vi "AudioStreamer.Initialize.vi"(1 "visible":bool) -> (0 "success":bool)   [LabVIEW 2020]
uses:
  <vilib>/Utility/sysdir.llb/System Directory Type.ctl
  <vilib>/Utility/config.llb/Read Key (I32).vi
  <vilib>/Utility/config.llb/NI_LVConfig.lvlib
panel:
  out "error out":errorcluster
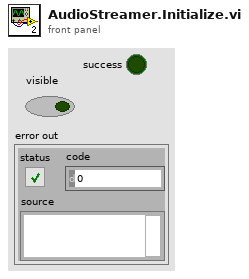
[diagram p1: front panel]
types:
  T1 = enum32{"Bad", "Idle", "Run top level", "Running"}
  T2 = enum32{"Invalid", "Standard", "Closed", "Hidden", "Minimized", "Maximized"}
  T3 = typedef "System Directory Type.ctl" = i32
  T4 = typedef "NI_LVConfig.lvlib/Config Data RefNum.ctl" = refnum<k1>
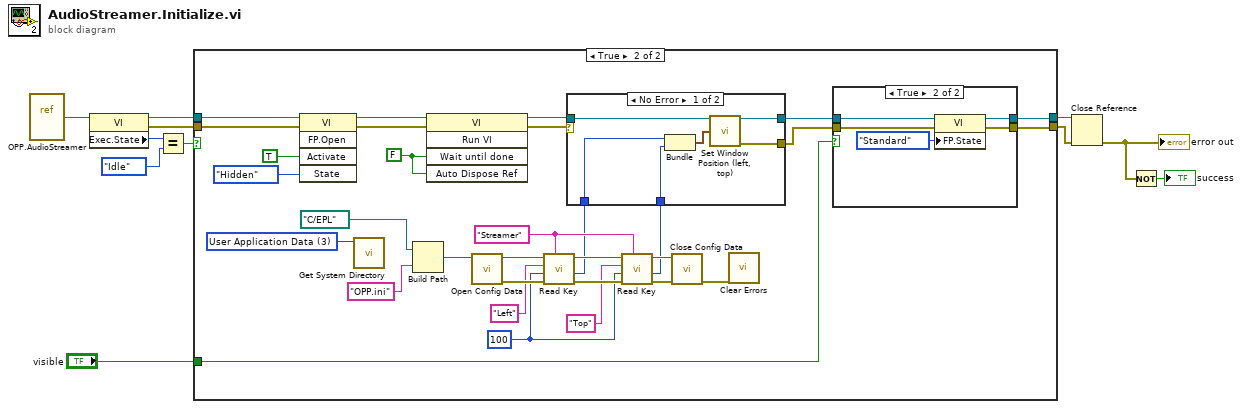
[diagram p0: block diagram]
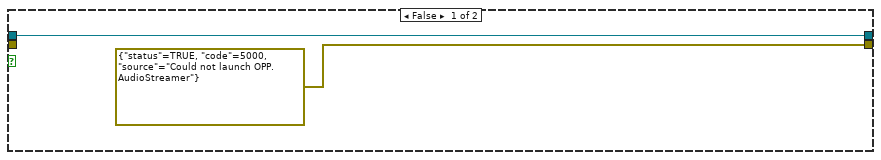
[diagram p2: hidden frame]
diagram:
  n1 = vi-ref "OPP.AudioStreamer.vi"() -> (w6:refnum<vi>)
  n2 = property class="VI"(reference=w6) -> (reference out=w11:refnum<vi>, error out=w10:errorcluster, "Exec.State"=w5:T1)  [unwired: 1 in]
  n3 = Equal?(x=w5, y=T1."Idle" ("Execution:State")) -> (x = y?=w4:bool)
  n4 = case shown="True" w4 {
    tunnel: w11 -> [w13 w43]
    tunnel: w10 -> [_ w42]
    tunnel: [w13 w16] -> w9
    tunnel: [errorcluster {"status"=TRUE, "code"=5000, "source"="Could not launch OPP.AudioStreamer"} ("error out") w15] -> w8
    tunnel: "visible" -> [_ w14]
    frame False {
    }
    frame True {
      w25 = 100 ("default value")
      w30 = "Streamer" ("section")
      w26 = T3 3 items=["User Home"=0, "User Desktop"=1, "User Documents"=2, "User Application Data"=3, "User Preferences"=4, "User Temporary"=5, "Public Documents"=6, "Public Application Data"=7, "Public Preferences"=8, "Public Cache"=13, "System Core Libraries"=9, "System Installed Libraries"=10, "Application Files"=11, "Boot Volume Root"=12] ("system directory type")
      w44 = FALSE ("Wait Until Done")
      n5 = invoke class="VI" method="FP.Open"(reference=w43, error in=w42, "Activate"=TRUE ("Activate?"), "State"=T2."Hidden" ("f")) -> (reference out=w40:refnum<vi>, error out=w39:errorcluster)  [unwired: 1 in, 3 out]
      n6 = call <vilib>:"Get System Directory.vi"("system directory type"=w26) -> ()  [unwired: 10 in, 1 out]
      n7 = Build Path(base path=path "C:/EPL", name or relative path="OPP.ini") -> (appended path=w37:path)
      n8 = invoke class="VI" method="Run VI"(reference=w40, error in=w39, "Wait until done"=w44, "Auto Dispose Ref"=w44) -> (reference out=w22:refnum<vi>, error out=w21:errorcluster)  [unwired: 1 in, 3 out]
      n9 = call <vilib>:"Open Config Data.vi"("configuration file path"=w37) -> ("error out"=w34:errorcluster, "refnum"=w36:T4)  [unwired: 8 in, 1 out]
      n10 = call-poly <vilib>:"Read Key.vi"("section"=w30, "error in (no error)"=w34, "default value"=w25, "key"="Left", "refnum"=w36) -> ("error out"=w33:errorcluster, "value"=w20:i32, "refnum out"=w35:T4)  [unwired: 3 in, 1 out]
      n11 = call-poly <vilib>:"Read Key.vi"("section"=w30, "error in (no error)"=w33, "default value"=w25, "key"="Top", "refnum"=w35) -> ("error out"=w32:errorcluster, "value"=w19:i32, "refnum out"=w31:T4)  [unwired: 3 in, 1 out]
      n12 = case shown="No Error" w21 {
        selector: w21 -> [_ w58]
        tunnel: w22 -> [w57 w59]
        tunnel: w20 -> [w56 _]
        tunnel: w19 -> [w55 _]
        tunnel: [w53 w59] -> w18
        tunnel: [w52 w58] -> w17
        frame No Error {
          n13 = Bundle("value"=w56, "value"=w55) -> (w54:cluster{"value":i32, "value":i32})  [unwired: 1 in]
          n14 = call "Set Window Position (left, top).vi"("VI in"=w57, "Coords"=w54) -> ("VI out"=w53:refnum<vi>, "error out"=w52:errorcluster)  [unwired: 12 in]
        }
        frame Error {
        }
      }
      n15 = call <vilib>:"Close Config Data.vi"("error in (no error)"=w32, "refnum"=w31) -> ("error out"=w24:errorcluster)  [unwired: 8 in, 1 out]
      n16 = call <vilib>:"Clear Errors.vi"("error in (no error)"=w24) -> ()  [unwired: 5 in, 2 out]
      n17 = case shown="True" w14 {
        tunnel: w18 -> [w46 w51]
        tunnel: w17 -> [w45 w50]
        tunnel: [w46 w49] -> w16
        tunnel: [w45 w48] -> w15
        frame False {
        }
        frame True {
          n18 = property class="VI"(reference=w51, error in=w50, "FP.State"=T2."Standard" ("Front Panel Window:State")) -> (reference out=w49:refnum<vi>, error out=w48:errorcluster)
        }
      }
    }
  }
  n19 = Close Reference(reference=w9, error in (no error)=w8) -> (error out=w2:errorcluster)
  "error out" <- w2
  n20 = Not(x=w2) -> (.not. x?=→"success":bool)
